vi "microsope.vi"(8 "Amplitude":u16(ring) items=["Channel 1", "Channel 2", "Channel 3", "Channel 4", "Math"], 9 "stop":bool, 10 "Source":u16(ring) items=["Channel 1", "Channel 2", "Channel 3", "Channel 4", "Math"], 11 "VISA Resource Name":refnum<visa-resource-name>="USB0::0x0957::0x1724::MY50340116::INSTR") -> (1 "Amplitude (mV)":dbl)   [LabVIEW 2015]
uses:
  <vilib>/Waveform/WDTFileIO.llb/Export Waveform To Spreadsheet File.vi
panel:
  in  "Sample frequency (KHz)":i8=2
  out "error out":errorcluster
  in  "# Points (Stop/Single required for >1k)":u16(ring)=3 items=["8M (Single required)", "4M", "2M", "1M", "500k", "200k", "100k", "50k", "20k", "10k", "5k", "2k", "1k", "500", "250", "100"]
  out "# Points":i32
  in  "Timeout Value (ms)":u32=2000
  in  "Create CSV Output File":bool
  in  "Output File":path
  out "Waveform Data":waveform(dbl)(graph)
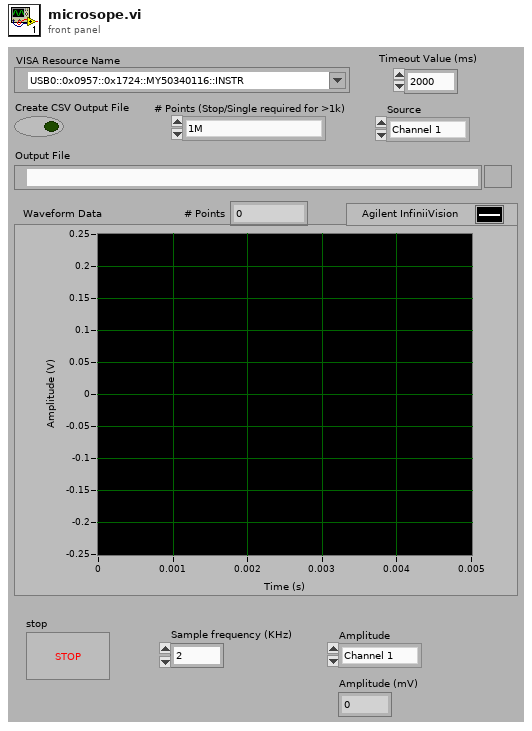
[diagram p1: front panel]
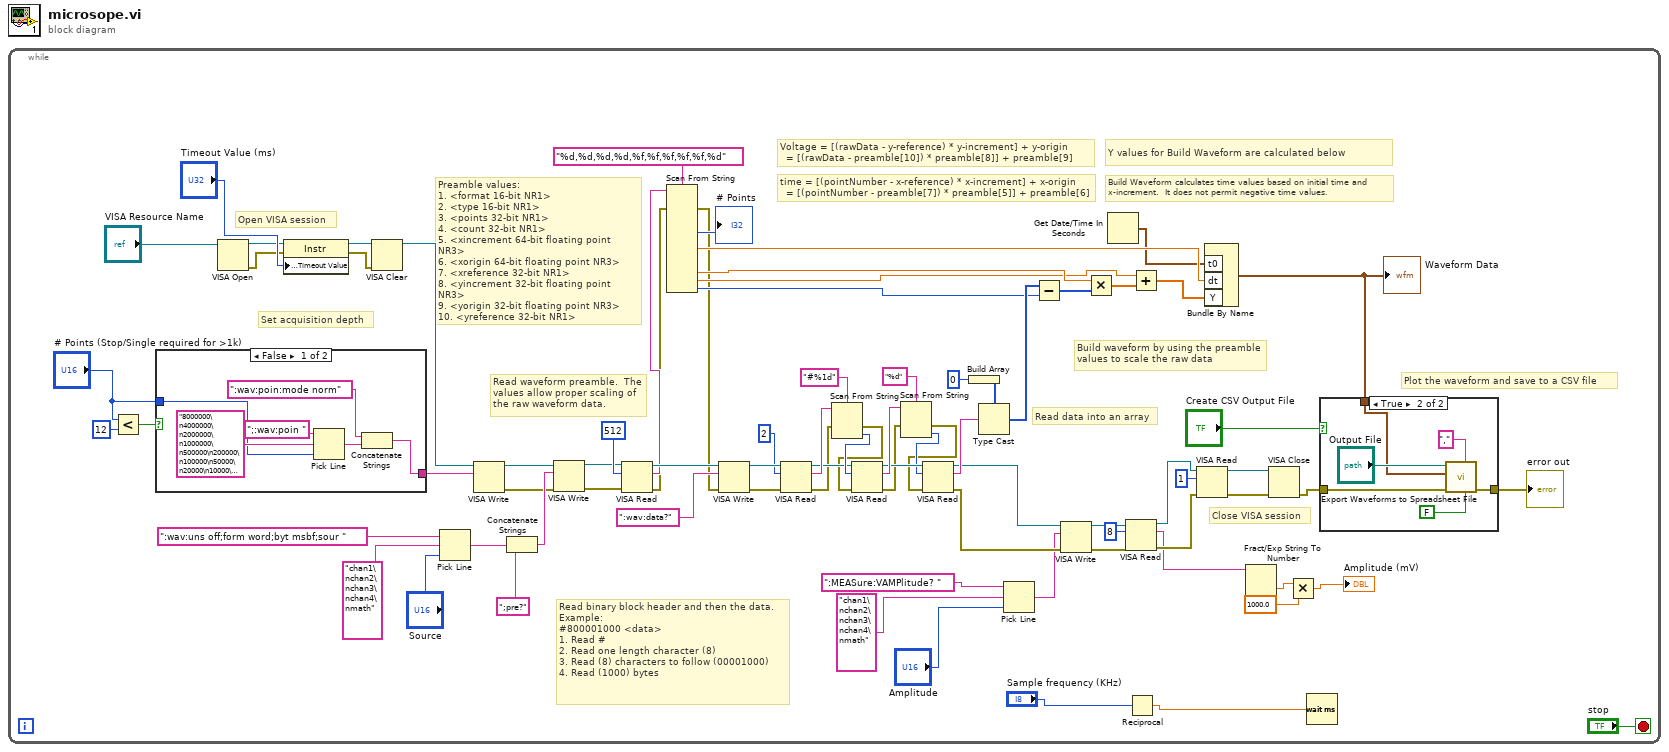
[diagram p0: block diagram]
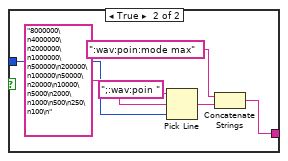
[diagram p2: hidden frame]
diagram:
  n1 = while {
    stop <- "stop" stop-if-true
    # "Close VISA session"
    # "Open VISA session"
    # "Set acquisition depth"
    # "Plot the waveform and save to a CSV file"
    # "Build Waveform calculates time values based on initial time and x-increment.  It does not permit negative time values."
    # "Y values for Build Waveform are calculated below"
    # "Build waveform by using the preamble values to scale the raw data"
    # "Read data into an array"
    # "Read binary block header and then the data.  Example: \n#800001000 <data>\n1. Read #\n2. Read one length character (8)\n3. Read (8) characters to follow (00001000)\n4. Read (1000) bytes"
    # "Read waveform preamble.  The values allow proper scaling of the raw waveform data."
    # "time = [(pointNumber - x-reference) * x-increment] + x-origin\n\t = [(pointNumber - preamble[7]) * preamble[5]] + preamble[6]"
    # "Voltage = [(rawData - y-reference) * y-increment] + y-origin\n\t\t= [(rawData - preamble[10]) * preamble[8]] + preamble[9]"
    # "Preamble values: \n1. <format 16-bit NR1>\n2. <type 16-bit NR1>\n3. <points 32-bit NR1>\n4. <count 32-bit NR1>\n5. <xincrement 64-bit floating point NR3>\n6. <xorigin 64-bit floating point NR3>\n7. <xreference 32-bit NR1>\n8. <yincrement 32-bit floating point NR3>\n9. <yorigin 32-bit floating point NR3>\n10. <yreference 32-bit NR1>"
    n2 = Less?(x="# Points (Stop/Single required for >1k)", y=u16 12) -> (x < y?=w27:bool)
    n3 = case shown="False" w27 {
      tunnel: [w84 w88] -> w32
      tunnel: "# Points (Stop/Single required for >1k)" -> [w85 w89]
      frame False {
        n4 = Pick Line(string ("")=";:wav:poin ", multi-line string="8000000\n4000000\n2000000\n1000000\n500000\n200000\n100000\n50000\n20000\n10000\n5000\n2000\n1000\n500\n250\n100\n", line index=w85) -> (output string=w83:string)
        n5 = Concatenate Strings(":wav:poin:mode norm" ("string"), w83) -> (w84:string)
      }
      frame True {
        n6 = Pick Line(string ("")=";:wav:poin ", multi-line string="8000000\n4000000\n2000000\n1000000\n500000\n200000\n100000\n50000\n20000\n10000\n5000\n2000\n1000\n500\n250\n100\n", line index=w89) -> (output string=w92:string)
        n7 = Concatenate Strings(":wav:poin:mode max" ("string"), w92) -> (w88:string)
      }
    }
    n8 = VISA Open(VISA resource name="VISA Resource Name") -> (VISA resource name=w37:refnum<visa-resource-name>, error out=w36:errorcluster)  [unwired: 4 in]
    n9 = property class="Instr"(reference=w37, error in=w36, "General Settings:Timeout Value"="Timeout Value (ms)") -> (reference out=w35:refnum<visa-resource-name>, error out=w34:errorcluster)
    n10 = VISA Clear(VISA resource name=w35, error in (no error)=w34) -> (VISA resource name out=w31:refnum<visa-resource-name>)  [unwired: 1 out]
    n11 = Pick Line(string ("")=":wav:uns off;form word;byt msbf;sour ", multi-line string="chan1\nchan2\nchan3\nchan4\nmath", line index="Source") -> (output string=w77:string)
    n12 = VISA Write(VISA resource name=w31, write buffer=w32) -> (VISA resource name out=w30:refnum<visa-resource-name>, error out=w29:errorcluster)  [unwired: 1 in, 1 out]
    n13 = Concatenate Strings(w77, ";pre?" ("string")) -> (w78:string)
    n14 = VISA Write(VISA resource name=w30, write buffer=w78, error in (no error)=w29) -> (VISA resource name out=w74:refnum<visa-resource-name>, error out=w73:errorcluster)  [unwired: 1 out]
    n15 = VISA Read(VISA resource name=w74, byte count=u32 512, error in (no error)=w73) -> (VISA resource name out=w72:refnum<visa-resource-name>, read buffer=w49:string, error out=w25:errorcluster)  [unwired: 1 out]
    n16 = Scan From String(format string="%d,%d,%d,%d,%f,%f,%f,%f,%f,%d", input string=w49, error in=w25) -> (error out=w24:errorcluster, output 3=→"# Points":i32, output 5=w42:dbl, output 8=w54:dbl, output 9=w52:dbl, output 10=w47:i32)  [unwired: 16 in, 2 out]
    n17 = VISA Write(VISA resource name=w72, write buffer=":wav:data?", error in (no error)=w24) -> (VISA resource name out=w70:refnum<visa-resource-name>, error out=w69:errorcluster)  [unwired: 1 out]
    n18 = VISA Read(VISA resource name=w70, byte count=u32 2, error in (no error)=w69) -> (VISA resource name out=w64:refnum<visa-resource-name>, read buffer=w67:string, error out=w23:errorcluster)  [unwired: 1 out]
    n19 = Scan From String(format string="#%1d", input string=w67, error in=w23) -> (error out=w22:errorcluster, output 1=w65:i32)  [unwired: 2 in, 2 out]
    n20 = VISA Read(VISA resource name=w64, byte count=w65, error in (no error)=w22) -> (VISA resource name out=w61:refnum<visa-resource-name>, read buffer=w63:string, error out=w21:errorcluster)  [unwired: 1 out]
    n21 = Scan From String(format string="%d", input string=w63, error in=w21) -> (error out=w20:errorcluster, output 1=w60:i32)  [unwired: 2 in, 2 out]
    n22 = VISA Read(VISA resource name=w61, byte count=w60, error in (no error)=w20) -> (VISA resource name out=w15:refnum<visa-resource-name>, read buffer=w57:string, error out=w12:errorcluster)  [unwired: 1 out]
    n23 = Build Array(i16 0 ("element")) -> (w58:i16[])
    n24 = Type Cast(type=w58, x=w57) -> (*(type *) &x=w48:i16[])
    n25 = Pick Line(string ("")=":MEASure:VAMPlitude? " ("write buffer"), multi-line string="chan1\nchan2\nchan3\nchan4\nmath", line index="Amplitude") -> (output string=w9:string)
    n26 = Subtract(x=w48, y=w47) -> (x-y=w55:i32[])
    n27 = VISA Write(VISA resource name=w15, write buffer=w9, error in (no error)=w12) -> (VISA resource name out=w14:refnum<visa-resource-name>, error out=w11:errorcluster)  [unwired: 1 out]
    n28 = Multiply(x=w54, y=w55) -> (x*y=w53:dbl[])
    n29 = Get Date/Time In Seconds() -> (seconds since 1Jan1904=w41:timestamp)
    n30 = VISA Read(VISA resource name=w14, byte count=u32 8, error in (no error)=w11) -> (VISA resource name out=w13:refnum<visa-resource-name>, read buffer=w4:string, error out=w10:errorcluster)  [unwired: 1 out]
    n31 = Reciprocal(x="Sample frequency (KHz)") -> (1/x=w16:dbl)
    n32 = Add(x=w52, y=w53) -> (x+y=w46:dbl[])
    n33 = VISA Read(VISA resource name=w13, byte count=u32 1, error in (no error)=w10) -> (VISA resource name out=w51:refnum<visa-resource-name>, error out=w50:errorcluster)  [unwired: 2 out]
    n34 = Bundle By Name("t0"=w41, "dt"=w42, "Y"=w46) -> (w40:waveform(dbl))  [unwired: 1 in]
    "Waveform Data" <- w40
    n35 = Fract/Exp String To Number(string=w4) -> (number=w3:dbl)  [unwired: 3 in, 1 out]
    n36 = VISA Close(VISA resource name=w51, error in (no error)=w50) -> (error out=w43:errorcluster)
    n37 = Multiply(x=w3, y=1000.0) -> (x*y=→"Amplitude (mV)":dbl)
    n38 = Wait (ms)(milliseconds to wait=w16) -> ()  [unwired: 1 out]
    n39 = case shown="True" "Create CSV Output File" {
      tunnel: w40 -> [_ w98]
      tunnel: w43 -> [w94 w97]
      tunnel: [w94 w95] -> w19
      frame False {
      }
      frame True {
        n40 = call-poly <vilib>:"Export Waveforms to Spreadsheet File.vi"("header? (write header:T)"=FALSE, "delimiter (Tab)"=",", "error in (no error)"=w97, "waveform"=w98, "file path (dialog if empty)"="Output File") -> ("error out"=w95:errorcluster)  [unwired: 5 in, 1 out]
      }
    }
    "error out" <- w19
  }
